vi "Stop Core.vi"(10 "final error code":i32, 11 "Analog Reader in":refnum<class "Analog Reader.lvclass">) -> (3 "Analog Reader out":refnum<class "Analog Reader.lvclass">)   [LabVIEW 2024, in "DAQmx Actor.lvlib" / "Analog Reader.lvclass"]
doc: "<p>(<strong>Filename</strong>: <span class=\"dnl\">Actor Framework.lvlib:Actor.lvclass:Stop Core.vi</span>)</p>\n<p>Defines what the actor does before it stops. Use the <strong>final error code</strong> input to determine whether the actor shut down in response to an error.</p>\n<p>By default, this method passes the Stop message along to all <a href=\"nihelplauncher://docs/csh?context=lvcore_lvcomm_af_launch_nested_actor\">auto-stop nested actors</a>. A descendant class may override this method to define additional behavior, such as shutting down any processes the actor initiated in its override of the <a href=\"nihelplauncher://docs/csh?context=lvcore_lvcomm_af_actor_core\">Actor Core</a> method.</p>"
uses:
  Analog Reader.lvclass
  Analog Reader.lvclass/Analog Reader.ctl
  DAQmx Actor/DAQmx Actor.lvclass
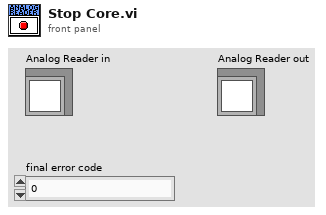
[diagram p1: front panel]
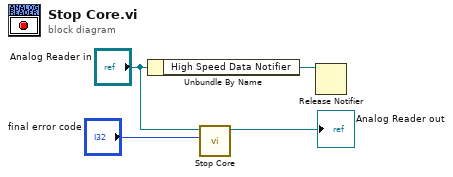
[diagram p0: block diagram]
diagram:
  n1 = Unbundle By Name("Analog Reader in") -> ("High Speed Data Notifier"=w1:refnum<notifier>)
  n2 = call-parent "Stop Core.vi"("final error code"="final error code", "DAQmx Actor in"="Analog Reader in") -> ("DAQmx Actor out"=→"Analog Reader out":refnum<class "Analog Reader.lvclass">)  [unwired: 9 in]
  n3 = Release Notifier(notifier=w1) -> ()  [unwired: 2 in, 3 out]
